vi "FT10_Semi-Auto Set Config.vi"(7 "Wait Time (ms)":i32=10, 9 "Mode in":T1, 10 "Port in":T2) -> (1 "Mode out":T1, 2 "Port out":T2, 3 "output cluster":T3)   [LabVIEW 2024]
doc: "Creates message for Message Handling Loop to set relay configuration for upcoming port activation."
uses:
  Controls/Control_Command Cluster.ctl
  Controls/Control_Semi-Auto Port.ctl
  Controls/Control_Semi-Auto Mode.ctl
  Controls/Control_PXI-7854R Set Config Cluster.ctl
  Controls/Control_PXI-7854R Set Config Enum.ctl
  Controls/Control_PXI-7854R Set Config Bool.ctl
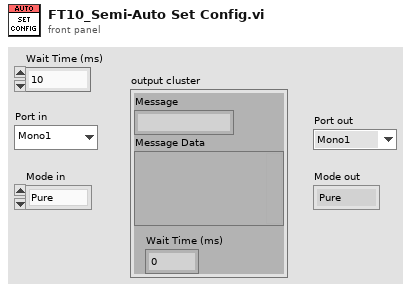
[diagram p1: front panel]
types:
  T1 = typedef "Control_Semi-Auto Mode.ctl" = enum16{"Pure", "Blend", "Spray", "Fulgerate", "Standard", "Macro", "Precision", "Ligasure", "Error"}
  T2 = typedef "Control_Semi-Auto Port.ctl" = enum16{"Mono1", "Mono2", "Bipolar", "Ligasure", "Error"}
  T3 = typedef "Control_Command Cluster.ctl" = cluster{"Message":string, "Message Data":variant, "Wait Time (ms)":i32}
  T4 = typedef "Control_PXI-7854R Set Config Bool.ctl" = bool
  T5 = typedef "Control_PXI-7854R Set Config Enum.ctl" = enum16{"Mono 1", "Mono 2", "BiPolar", "LigaSure", "Off"}
  T6 = typedef "Control_PXI-7854R Set Config Cluster.ctl" = cluster{"7854 Config Enum":T5, "7854 Set Config":T4}
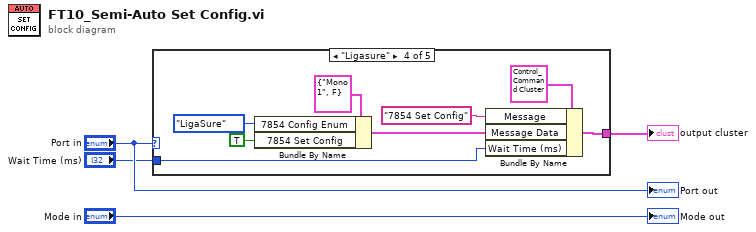
[diagram p0: block diagram]
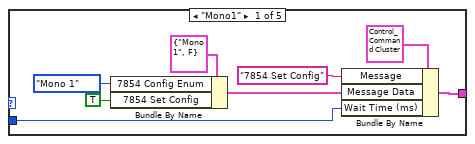
[diagram p2: hidden frame]
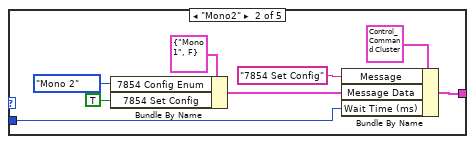
[diagram p3: hidden frame]
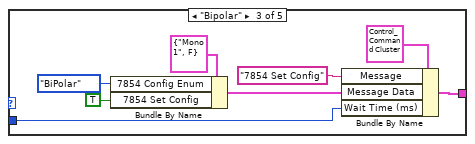
[diagram p4: hidden frame]
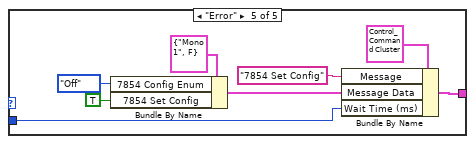
[diagram p5: hidden frame]
diagram:
  n1 = case shown="\"Ligasure\"" "Port in" {
    tunnel: [w6 w14 w22 w30 w38] -> w3
    tunnel: "Wait Time (ms)" -> [w5 w13 w21 w29 w37]
    frame "Mono1" {
      n2 = Bundle By Name(cluster=T6 {"7854 Config Enum"=enum."Mono 1", "7854 Set Config"=FALSE}, "7854 Config Enum"=Control_PXI-7854R_Set_Config_Enum."Mono 1", "7854 Set Config"=T4 TRUE) -> (w7:T6)
      n3 = Bundle By Name(cluster=T3 {"Message"="", "Message Data"=variant, "Wait Time (ms)"=0}, "Message"="7854 Set Config", "Message Data"=w7, "Wait Time (ms)"=w5) -> (w6:T3)
    }
    frame "Mono2" {
      n4 = Bundle By Name(cluster=T6 {"7854 Config Enum"=enum."Mono 1", "7854 Set Config"=FALSE}, "7854 Config Enum"=Control_PXI-7854R_Set_Config_Enum."Mono 2", "7854 Set Config"=T4 TRUE) -> (w15:T6)
      n5 = Bundle By Name(cluster=T3 {"Message"="", "Message Data"=variant, "Wait Time (ms)"=0}, "Message"="7854 Set Config", "Message Data"=w15, "Wait Time (ms)"=w13) -> (w14:T3)
    }
    frame "Bipolar" {
      n6 = Bundle By Name(cluster=T6 {"7854 Config Enum"=enum."Mono 1", "7854 Set Config"=FALSE}, "7854 Config Enum"=Control_PXI-7854R_Set_Config_Enum."BiPolar", "7854 Set Config"=T4 TRUE) -> (w23:T6)
      n7 = Bundle By Name(cluster=T3 {"Message"="", "Message Data"=variant, "Wait Time (ms)"=0}, "Message"="7854 Set Config", "Message Data"=w23, "Wait Time (ms)"=w21) -> (w22:T3)
    }
    frame "Ligasure" {
      n8 = Bundle By Name(cluster=T6 {"7854 Config Enum"=enum."Mono 1", "7854 Set Config"=FALSE}, "7854 Config Enum"=Control_PXI-7854R_Set_Config_Enum."LigaSure", "7854 Set Config"=T4 TRUE) -> (w31:T6)
      n9 = Bundle By Name(cluster=T3 {"Message"="", "Message Data"=variant, "Wait Time (ms)"=0}, "Message"="7854 Set Config", "Message Data"=w31, "Wait Time (ms)"=w29) -> (w30:T3)
    }
    frame "Error" {
      n10 = Bundle By Name(cluster=T6 {"7854 Config Enum"=enum."Mono 1", "7854 Set Config"=FALSE}, "7854 Config Enum"=Control_PXI-7854R_Set_Config_Enum."Off", "7854 Set Config"=T4 TRUE) -> (w39:T6)
      n11 = Bundle By Name(cluster=T3 {"Message"="", "Message Data"=variant, "Wait Time (ms)"=0}, "Message"="7854 Set Config", "Message Data"=w39, "Wait Time (ms)"=w37) -> (w38:T3)
    }
  }
  "output cluster" <- w3
  "Port out" <- "Port in"
  "Mode out" <- "Mode in"
